vi "Calculate Delay.vi"(8 "error in (no error)":errorcluster, 11 "Readout Charact in":refnum<class "Readout Charact.lvclass">) -> (0 "error out":errorcluster, 3 "Readout Charact out":refnum<class "Readout Charact.lvclass">)   [LabVIEW 2018, in "Readout Charact.lvclass"]
uses:
  Readout Charact.lvclass
  Readout Charact.lvclass/Readout Charact.ctl
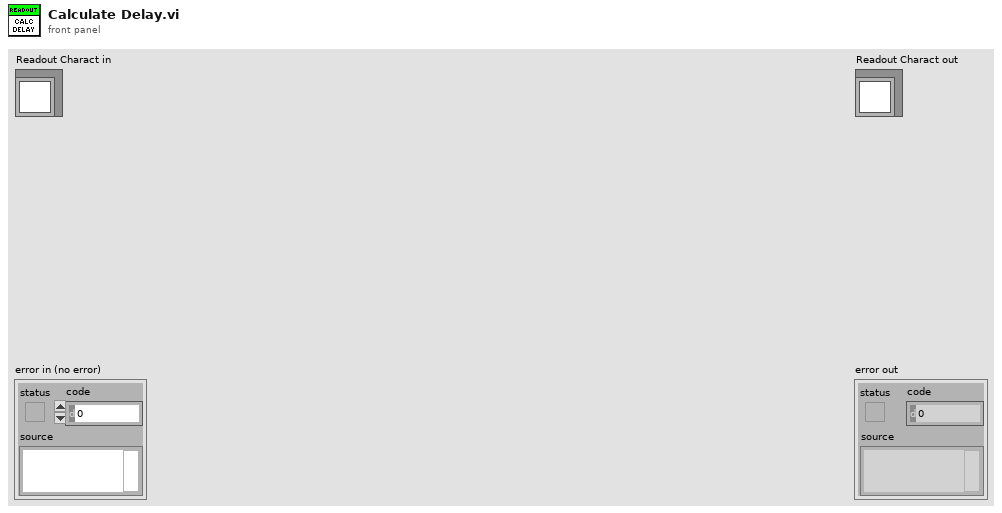
[diagram p1: front panel]
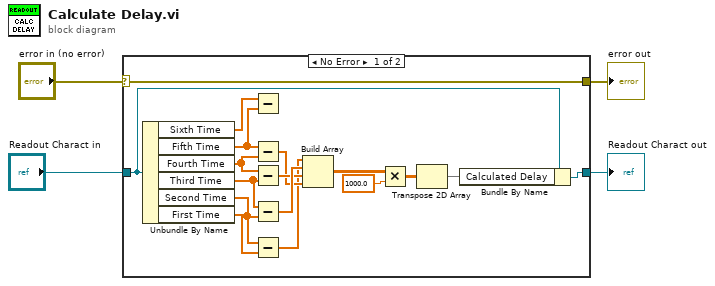
[diagram p0: block diagram]
diagram:
  n1 = case shown="No Error" "error in (no error)" {
    selector: "error in (no error)" -> [w21 w23]
    tunnel: [w21 w23] -> w3
    tunnel: [w16 w22] -> w1
    tunnel: "Readout Charact in" -> [w15 w22]
    frame No Error {
      n2 = Unbundle By Name(w15) -> ("Sixth Time"=w10:dbl[], "Fifth Time"=w9:dbl[], "Fourth Time"=w20:dbl[], "Third Time"=w19:dbl[], "Second Time"=w18:dbl[], "First Time"=w17:dbl[])
      n3 = Subtract(x=w10, y=w9) -> ()  [unwired: 1 out]
      n4 = Subtract(x=w9, y=w20) -> (x-y=w11:dbl[])
      n5 = Subtract(x=w20, y=w19) -> (x-y=w13:dbl[])
      n6 = Subtract(x=w19, y=w18) -> (x-y=w14:dbl[])
      n7 = Subtract(x=w18, y=w17) -> (x-y=w8:dbl[])
      n8 = Build Array(w8, w14, w13, w11) -> (w7:dbl[][])
      n9 = Multiply(x=w7, y=1000.0) -> (x*y=w6:dbl[][])
      n10 = Transpose 2D Array(2D array=w6) -> (transposed array=w5:dbl[][])
      n11 = Bundle By Name(cluster=w15, "Calculated Delay"=w5) -> (w16:refnum<class "Readout Charact.lvclass">)
    }
    frame Error {
    }
  }
  "error out" <- w3
  "Readout Charact out" <- w1
